vi "Generate Error.vi"(8 "error in (no error)":errorcluster, 11 "modbus in":refnum<class "libmodbus.lvclass">) -> (0 "error out":errorcluster, 3 "modbus out":refnum<class "libmodbus.lvclass">)   [LabVIEW 2017, in "libmodbus.lvlib" / "libmodbus.lvclass"]
doc: "Generates an error from the actual errno."
uses:
  libmodbus.lvclass
  libmodbus.lvclass/libmodbus.ctl
  Utilities/Utilities.lvlib
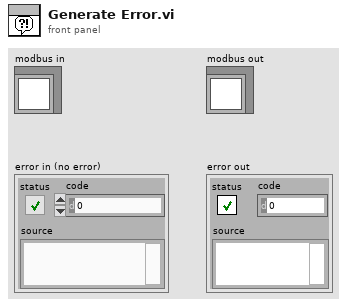
[diagram p1: front panel]
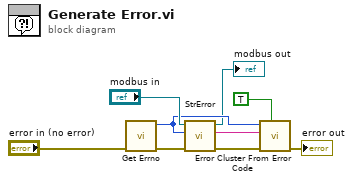
[diagram p0: block diagram]
diagram:
  n1 = call "Get Errno.vi"("error in (no error)"="error in (no error)") -> ("error out"=w9:errorcluster, "errno"=w5:u32)  [unwired: 9 in]
  n2 = call "StrError.vi"("error in (no error)"=w9, "errnum"=w5, "modbus in"="modbus in") -> ("error out"=w6:errorcluster, "error message"=w4:string, "modbus out"=→"modbus out":refnum<class "libmodbus.lvclass">)  [unwired: 6 in]
  n3 = call <vilib>:"Error Cluster From Error Code.vi"("show call chain? (False)"=TRUE, "error in (no error)"=w6, "error message (\"\")"=w4, "error code (0)"=w5) -> ("error out"=→"error out":errorcluster)  [unwired: 5 in]
